vi "Close_Instr.vi"(8 "error in (no error)":errorcluster caption="entrée d'erreur (pas d'erreur)", 11 "Class Instrument Power_Supply en entrée":refnum<class "Class Instrument Power_Supply.lvclass">) -> (0 "error out":errorcluster caption="sortie d'erreur", 3 "Class Instrument Power_Supply en sortie":refnum<class "Class Instrument Power_Supply.lvclass">)   [LabVIEW 2020, in "Library Instrument & Equipement.lvlib" / "Library Instruments.lvlib" / "Class Instrument Power_Supply.lvclass"]
uses:
  Class Instrument Power_Supply.lvclass
  Class Instrument Power_Supply.lvclass/Class Instrument Power_Supply.ctl
  Power_Supply/Power_Supply (Default)/Power_Supply (Default).lvclass
  Instrument (Default)/Class Instrument (Default).lvclass
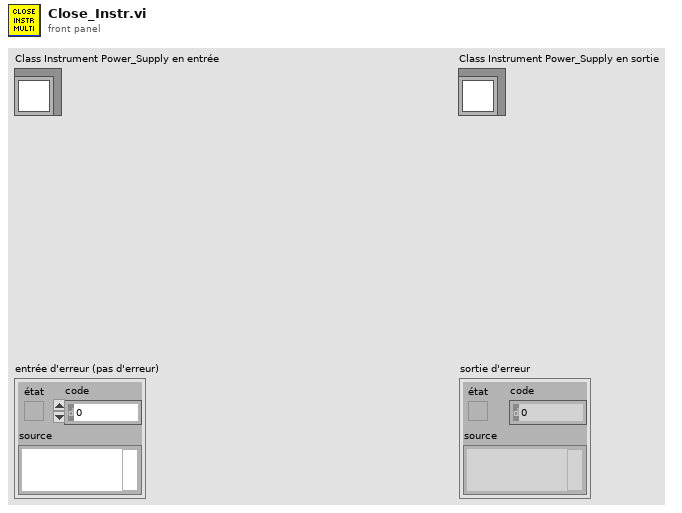
[diagram p1: front panel]
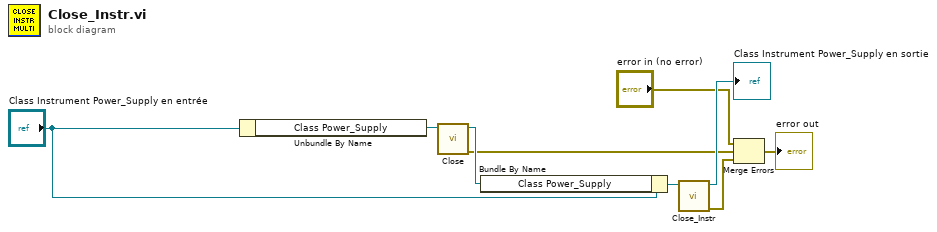
[diagram p0: block diagram]
diagram:
  n1 = Unbundle By Name("Class Instrument Power_Supply en entrée") -> ("Class Power_Supply"=w9:refnum<class "Power_Supply (Default).lvclass">)
  n2 = call-dynamic "Close.vi"("Power_Supply (Default) en entrée"=w9) -> ("error out"=w3:errorcluster, "Power_Supply (Default) en sortie"=w8:refnum<class "Power_Supply (Default).lvclass">)  [unwired: 9 in]
  n3 = Bundle By Name(cluster="Class Instrument Power_Supply en entrée", "Class Power_Supply"=w8) -> (w5:refnum<class "Class Instrument Power_Supply.lvclass">)
  n4 = call-parent "Close_Instr.vi"("Class Instrument (Default) en entrée"=w5) -> ("error out"=w2:errorcluster, "Class Instrument (Default) en sortie"=→"Class Instrument Power_Supply en sortie":refnum<class "Class Instrument Power_Supply.lvclass">)  [unwired: 9 in]
  n5 = Merge Errors("error in (no error)", w3, w2) -> (→"error out":errorcluster)
